vi "read data setting from xml.vi"(8 "error constant":errorcluster, 11 "DAQ Config in":T1) -> (0 "error out":errorcluster, 3 "DAQ Config out":T1)   [LabVIEW 2017]
uses:
  Control/Config chanel.ctl
  <vilib>/Utility/xml.llb/Read From XML File(string).vi
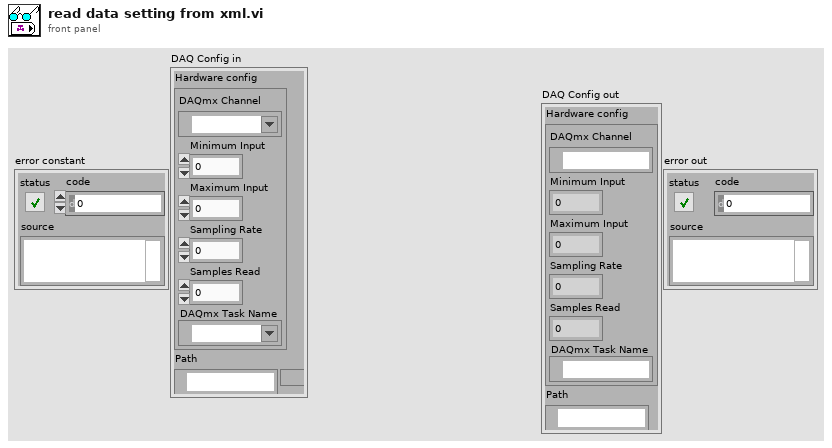
[diagram p1: front panel]
types:
  T1 = typedef "Config chanel.ctl" = cluster{"Hardware config":cluster{"DAQmx Channel":tag, "Minimum Input":dbl, "Maximum Input":dbl, "Sampling Rate":dbl, "Samples Read":dbl, "DAQmx Task Name":refnum<k21>}, "Path":path}
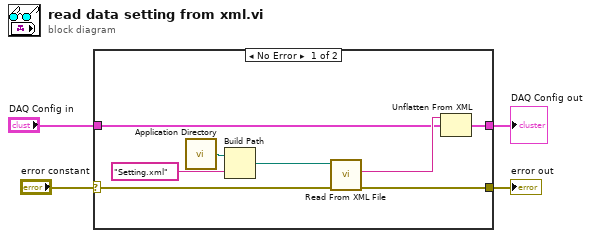
[diagram p0: block diagram]
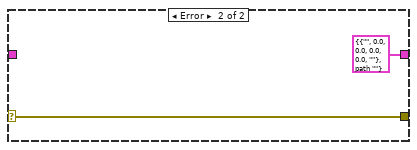
[diagram p2: hidden frame]
diagram:
  n1 = case shown="No Error" "error constant" {
    selector: "error constant" -> [w8 w14]
    tunnel: [w7 w14] -> w3
    tunnel: [w6 T1 {"Hardware config"={"DAQmx Channel"="", "Minimum Input"=0.0, "Maximum Input"=0.0, "Sampling Rate"=0.0, "Samples Read"=0.0, "DAQmx Task Name"=""}, "Path"=path ""} ("DAQ Config")] -> w2
    tunnel: "DAQ Config in" -> [w5 _]
    frame No Error {
      n2 = call <vilib>:"Application Directory.vi"() -> ("Application Directory"=w12:path)
      n3 = Build Path(base path=w12, name or relative path="Setting.xml") -> (appended path=w10:path)
      n4 = call-poly <vilib>:"Read From XML File.vi"("error in (no error)"=w8, "XML File Path"=w10) -> ("error out"=w7:errorcluster, "XML Elements"=w9:string)  [unwired: 7 in, 1 out]
      n5 = Unflatten From XML(xml string=w9, type=w5) -> (value=w6:T1)  [unwired: 1 in, 1 out]
    }
    frame Error {
    }
  }
  "error out" <- w3
  "DAQ Config out" <- w2
